vi "Load Subroutine Test Exec.vi"(4 "Path Builder":refnum<class "IPath Builder.lvclass">, 5 "Subroutine in":refnum<class "Subroutine.lvclass">, 6 "Persistence in":refnum<class "IPersist.lvclass">, 7 "Linked List ID":string, 8 "error in (no error)":errorcluster, 10 "Subroutine Path":path, 11 "Linked List Ref":refnum<data-value>) -> (0 "error out":errorcluster, 1 "Test File Version Match":bool, 2 "Test Executive Version Match":bool, 3 "Linked List Ref out":refnum<data-value>)   [LabVIEW 2017, in "Custom Type Test Executive.lvlib" / "Subroutine.lvclass"]
uses:
  <vilib>/gpm_packages/@cs/test-executive/Source/Custom Type Test Executive/Subroutine/Subroutine.lvclass
  <vilib>/gpm_packages/@cs/linked-list/Source/Linked List/ILinkedList/ILinked List.lvclass
  <vilib>/gpm_packages/@cs/persistence/source/IPersist/IPersist.lvclass
  <vilib>/gpm_packages/@cs/test-executive/Source/Path Builder/IPath Builder/IPath Builder.lvclass
  <vilib>/gpm_packages/@cs/test-executive/Source/Test Executive/ITestExecutive/ITest Executive.lvclass
  <vilib>/gpm_packages/@cs/test-executive/Source/Custom Type Test Executive/Test Executive Data Type/Test Executive.lvclass/Test Executive.ctl
  <vilib>/gpm_packages/@cs/data-type-serializer/source/Boolean/Boolean.lvclass/Boolean.ctl
  <vilib>/gpm_packages/@cs/test-executive/Source/Custom Type Test Executive/Custom Type Test Executive/Custom Type Test Executive.lvclass
  C:/Program Files/National Instruments/LabVIEW 2017/vi.lib/gpm_packages/@cs/test-executive/Source/Test Executive/ITestExecutive/ITest Executive.lvclass
  <vilib>/gpm_packages/@cs/data-type-serializer/source/String/String.lvclass/String.ctl
  8fd00299-f1f7-40b8-accc-d4ca8393805f.vi
  7c02b004-8b9d-45a5-be84-3e65cc974b1d.vi
  eeacede9-d011-4dba-942b-6df48e717fe6.vi
  82c2d36c-c725-40f4-a6f6-462dea4f116e.vi
  7a4b305b-7132-4b75-8629-811f3558ef42.vi
  cfb7364d-dae3-4f2b-ba87-61db7f054fd9.vi
  1f521296-bf4a-4187-b7fe-4ed0693accc0.vi
  b9c2613a-6aa9-4761-86d5-781f96568d67.vi
  <vilib>/gpm_packages/@cs/test-executive/Source/Custom Type Test Executive/Test Executive Data Type/Test Executive.lvclass
  C:/Program Files/National Instruments/LabVIEW 2017/vi.lib/gpm_packages/@cs/data-type-serializer/source/Data Type/Data Type.lvclass
  <vilib>/Utility/error.llb/Error Cluster From Error Code.vi
  <vilib>/gpm_packages/@cs/data-type-serializer/source/Boolean/Boolean.lvclass
  <vilib>/gpm_packages/@cs/data-type-serializer/source/String/String.lvclass
  <vilib>/gpm_packages/@cs/test-executive/Source/Test Executive/TestExecutive Ref/TestExecutive Ref.lvclass
  <vilib>/gpm_packages/@cs/linked-list/Source/Linked List/Linked List Ref/Linked List Ref.lvclass
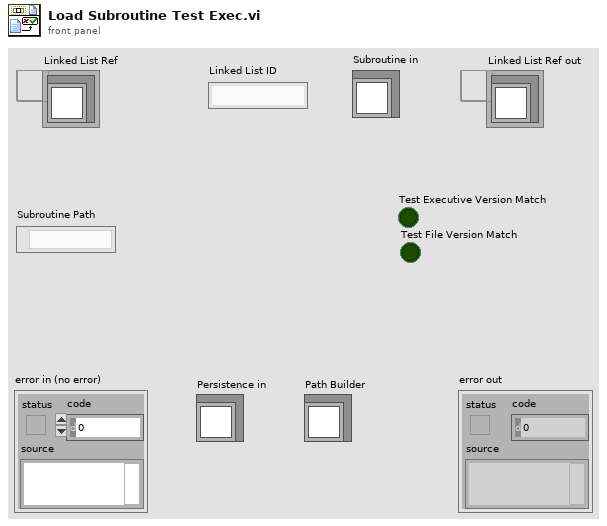
[diagram p1: front panel]
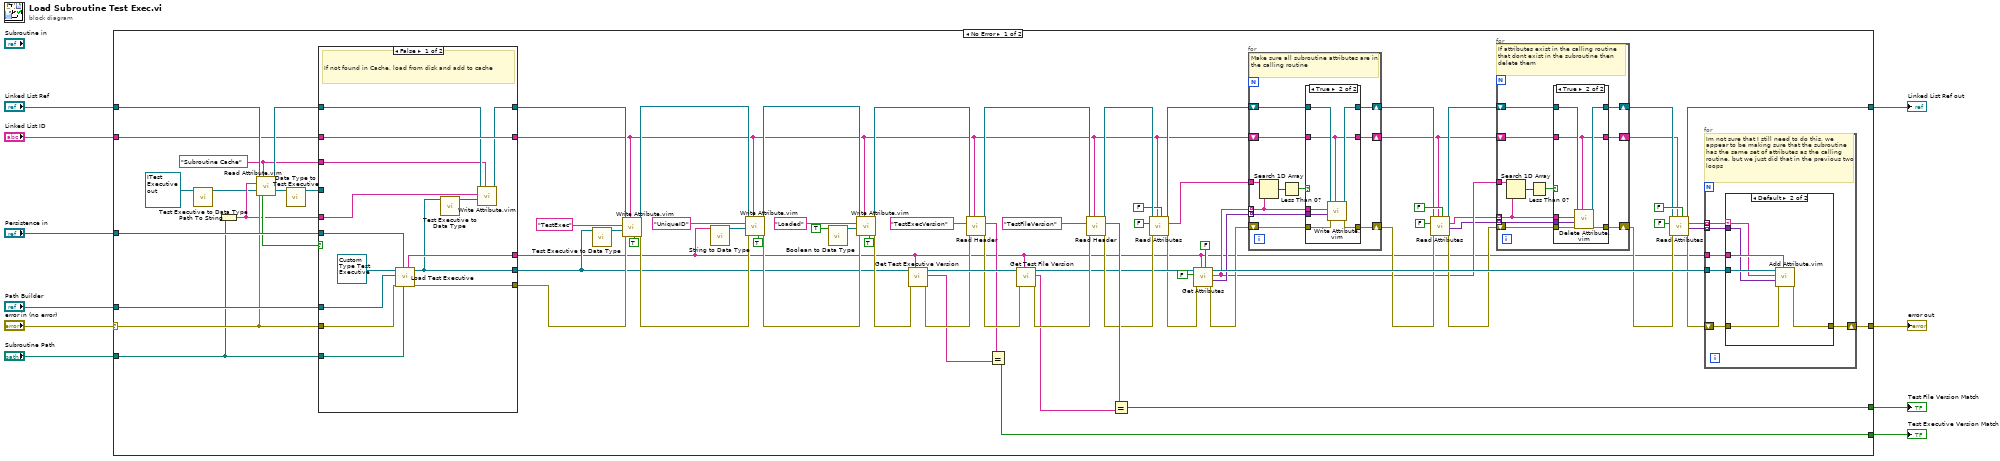
[diagram p0: block diagram]
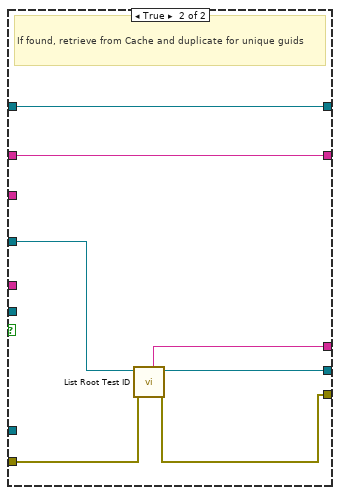
[diagram p2: hidden frame]
diagram:
  n1 = case shown="No Error" "error in (no error)" {
    selector: "error in (no error)" -> [w29 w168]
    tunnel: "Persistence in" -> [w82 _]
    tunnel: "Subroutine Path" -> [w28 _]
    tunnel: "Path Builder" -> [w81 _]
    tunnel: "Linked List Ref" -> [w30 w169]
    tunnel: [w65 _] -> w4
    tunnel: [w64 _] -> w3
    tunnel: "Linked List ID" -> [w24 _]
    tunnel: [w36 w169] -> w1
    tunnel: [w60 w168] -> w2
    frame No Error {
      w21 = "Subroutine Cache" ("Name")
      n2 = call <vilib>:"Test Executive to Data Type.vi"("Test Executive Ref"=refnum<data-value> refnum ("Test Executive Ref out")) -> ("Boolean out"=w19:refnum<class "Test Executive.lvclass">)  [unwired: 9 in, 1 out]
      n3 = Path To String(path=w28) -> (string=w22:string)
      n4 = call "Read Attribute.vim"("Linked List Ref"=w30, "Linked List ID"=w21, "Attribute Name"=w22, "Type"=w19, "error in (no error)"=w29) -> ("Linked List Ref out"=w26:refnum<data-value>, "Attribute"=w18:refnum<class "Test Executive.lvclass">, "Found?"=w27:bool)  [unwired: 5 in, 3 out]
      n5 = call <vilib>:"Data Type to Test Executive.vi"("Data Type"=w18) -> ("Test Executive Ref"=w17:refnum<data-value>)  [unwired: 9 in, 1 out]
      n6 = case shown="False" w27 {
        tunnel: [w105 w109] -> w87
        tunnel: w82 -> [w104 _]
        tunnel: w81 -> [w103 _]
        tunnel: [w94 w107] -> w15
        tunnel: [w95 w106] -> w13
        tunnel: w29 -> [w102 w110]
        tunnel: w28 -> [w101 _]
        tunnel: [w98 w112] -> w25
        tunnel: w26 -> [w99 w112]
        tunnel: [w100 w111] -> w23
        tunnel: w24 -> [w100 w111]
        tunnel: w22 -> [w96 _]
        tunnel: w21 -> [w97 _]
        tunnel: w17 -> [_ w108]
        frame False {
          # "If not found in Cache, load from disk and add to cache"
          n7 = call <vilib>:"Load Test Executive.vi"("Folder"=w101, "Persistence in"=w104, "error in (no error)"=w102, "Path Builder"=w103, "Test Executive"=refnum<class "Custom Type Test Executive.lvclass"> refnum ("Custom Type Test Executive.lvlib:Custom Type Test Executive.lvclass")) -> ("error out"=w105:errorcluster, "Test Executive Ref out"=w94:refnum<data-value>, "Root ID"=w95:string)  [unwired: 4 in]
          n8 = call <vilib>:"Test Executive to Data Type.vi"("Test Executive Ref"=w94) -> ("Boolean out"=w93:refnum<class "Test Executive.lvclass">)  [unwired: 9 in, 1 out]
          n9 = call "Write Attribute.vim"("Linked List ID"=w97, "Attribute"=w93, "Attribute Name"=w96, "Linked List Ref"=w99) -> ("Linked List Ref out"=w98:refnum<data-value>)  [unwired: 4 in, 3 out]
        }
        frame True {
          # "If found, retrieve from Cache and duplicate for unique guids"
          n10 = call <vilib>:"List Root Test ID.vi"("error in (no error)"=w110, "Test Executive Ref"=w108) -> ("error out"=w109:errorcluster, "Test Executive Ref out"=w107:refnum<data-value>, "Root ID"=w106:string)  [unwired: 5 in, 2 out]
        }
      }
      n11 = call <vilib>:"Test Executive to Data Type.vi"("Test Executive Ref"=w15) -> ("Boolean out"=w16:refnum<class "Test Executive.lvclass">)  [unwired: 9 in, 1 out]
      n12 = call "Write Attribute.vim"("Private?"=TRUE, "Linked List ID"=w23, "error in (no error)"=w87, "Attribute"=w16, "Attribute Name"="TestExec", "Linked List Ref"=w25) -> ("error out"=w88:errorcluster, "Linked List Ref out"=w80:refnum<data-value>)  [unwired: 2 in, 2 out]
      n13 = call <vilib>:"String to Data Type.vi"("String"=w13) -> ("Boolean out"=w14:refnum<class "String.lvclass">)  [unwired: 9 in, 1 out]
      n14 = call "Write Attribute.vim"("Private?"=TRUE, "Linked List ID"=w23, "error in (no error)"=w88, "Attribute"=w14, "Attribute Name"="UniqueID", "Linked List Ref"=w80) -> ("error out"=w84:errorcluster, "Linked List Ref out"=w79:refnum<data-value>)  [unwired: 2 in, 2 out]
      n15 = call <vilib>:"Boolean to Data Type.vi"("Boolean"=TRUE) -> ("Boolean out"=w12:refnum<class "Boolean.lvclass">)  [unwired: 9 in, 1 out]
      n16 = call "Write Attribute.vim"("Private?"=TRUE, "Linked List ID"=w23, "error in (no error)"=w84, "Attribute"=w12, "Attribute Name"="Loaded", "Linked List Ref"=w79) -> ("error out"=w77:errorcluster, "Linked List Ref out"=w76:refnum<data-value>)  [unwired: 2 in, 2 out]
      n17 = call <vilib>:"Get Test Executive Version.vi"("Unique ID"=w13, "error in (no error)"=w77, "Test Executive Ref"=w15) -> ("error out"=w74:errorcluster, "Test Executive Version"=w68:string, "Test Executive Ref out"=w78:refnum<data-value>)  [unwired: 5 in, 1 out]
      n18 = call <vilib>:"Read Header.vi"("Linked List ID"=w23, "error in (no error)"=w74, "Header Name"="TestExecVersion" ("String"), "Linked List Ref"=w76) -> ("error out"=w73:errorcluster, "Header Value"=w69:string, "Linked List Ref out"=w72:refnum<data-value>)  [unwired: 4 in, 1 out]
      n19 = Equal?(x=w69, y=w68) -> (x = y?=w65:bool)
      n20 = call <vilib>:"Get Test File Version.vi"("Unique ID"=w13, "error in (no error)"=w73, "Test Executive Ref"=w78) -> ("error out"=w71:errorcluster, "Test File Version"=w66:string, "Test Executive Ref out"=w58:refnum<data-value>)  [unwired: 5 in, 1 out]
      n21 = call <vilib>:"Read Header.vi"("Linked List ID"=w23, "error in (no error)"=w71, "Header Name"="TestFileVersion" ("String"), "Linked List Ref"=w72) -> ("error out"=w62:errorcluster, "Header Value"=w67:string, "Linked List Ref out"=w63:refnum<data-value>)  [unwired: 4 in, 1 out]
      n22 = Equal?(x=w67, y=w66) -> (x = y?=w64:bool)
      n23 = call <vilib>:"Read Attributes.vi"("Flatten Pointer?"=FALSE, "Linked List ID"=w23, "error in (no error)"=w62, "Include Private?"=FALSE, "Linked List Ref"=w63) -> ("error out"=w54:errorcluster, "Attribute Names out"=w53:string[], "Linked List Ref out"=w51:refnum<data-value>)  [unwired: 1 in, 3 out]
      n24 = call <vilib>:"Get Attributes.vi"("Flatten Pointer?"=FALSE, "Test ID"=w13, "error in (no error)"=w54, "Include Private?"=FALSE, "Test Executive Ref"=w58) -> ("error out"=w50:errorcluster, "Attributes"=w52:variant[], "Attribute Names out"=w42:string[], "Test Executive Ref out"=w57:refnum<data-value>)  [unwired: 1 in, 2 out]
      n25 = for {
        tunnel: w42 -> [w136] mode=indexing
        tunnel: w52 -> [w135] mode=indexing
        shift-right: [w141] -> w46
        shift-left: w51 -> [w142]
        tunnel: w53 -> [w143]
        shift-right: [w139] -> w47
        shift-left: w50 -> [w140]
        shift-right: [w134] -> w44
        shift-left: w23 -> [w138]
        # "Make sure all subroutine attributes are in the calling routine"
        n26 = Search 1D Array(1D array=w143, element=w136) -> (index of element=w144:i32)  [unwired: 1 in]
        n27 = Less Than 0?(x=w144) -> (x < 0?=w137:bool)
        n28 = case shown="True" w137 {
          tunnel: w142 -> [w147 w154]
          tunnel: [w147 w153] -> w141
          tunnel: w140 -> [w146 w152]
          tunnel: [w146 w151] -> w139
          tunnel: w138 -> [w145 w148]
          tunnel: w136 -> [_ w150]
          tunnel: w135 -> [_ w149]
          tunnel: [w145 w148] -> w134
          frame False {
          }
          frame True {
            n29 = call "Write Attribute.vim"("Linked List ID"=w148, "error in (no error)"=w152, "Attribute"=w149, "Attribute Name"=w150, "Linked List Ref"=w154) -> ("error out"=w151:errorcluster, "Linked List Ref out"=w153:refnum<data-value>)  [unwired: 3 in, 2 out]
          }
        }
      }
      n30 = call <vilib>:"Read Attributes.vi"("Flatten Pointer?"=FALSE, "Linked List ID"=w44, "error in (no error)"=w47, "Include Private?"=FALSE, "Linked List Ref"=w46) -> ("error out"=w43:errorcluster, "Attributes"=w40:variant[], "Attribute Names out"=w41:string[], "Linked List Ref out"=w45:refnum<data-value>)  [unwired: 1 in, 2 out]
      n31 = for {
        tunnel: w41 -> [w115] mode=indexing
        tunnel: w40 -> [w114] mode=indexing
        shift-right: [w120] -> w37
        shift-left: w45 -> [w121]
        tunnel: w42 -> [w122]
        shift-right: [w118] -> w34
        shift-left: w43 -> [w119]
        shift-right: [w113] -> w35
        shift-left: w44 -> [w117]
        # "If attributes exist in the calling routine that dont exist in the subroutine then delete them"
        n32 = Search 1D Array(1D array=w122, element=w115) -> (index of element=w123:i32)  [unwired: 1 in]
        n33 = Less Than 0?(x=w123) -> (x < 0?=w116:bool)
        n34 = case shown="True" w116 {
          tunnel: w121 -> [w126 w133]
          tunnel: [w126 w132] -> w120
          tunnel: w119 -> [w125 w130]
          tunnel: [w125 w129] -> w118
          tunnel: w117 -> [w124 w131]
          tunnel: w115 -> [_ w128]
          tunnel: w114 -> [_ w127]
          tunnel: [w124 w131] -> w113
          frame False {
          }
          frame True {
            n35 = call "Delete Attribute.vim"("Linked List ID"=w131, "error in (no error)"=w130, "Type"=w127, "Attribute Name"=w128, "Linked List Ref"=w133) -> ("error out"=w129:errorcluster, "Linked List Ref out"=w132:refnum<data-value>)  [unwired: 4 in, 1 out]
          }
        }
      }
      n36 = call <vilib>:"Read Attributes.vi"("Flatten Pointer?"=FALSE, "Linked List ID"=w35, "error in (no error)"=w34, "Include Private?"=FALSE, "Linked List Ref"=w37) -> ("error out"=w33:errorcluster, "Attributes"=w32:variant[], "Attribute Names out"=w31:string[], "Linked List Ref out"=w36:refnum<data-value>)  [unwired: 1 in, 2 out]
      n37 = for {
        tunnel: w57 -> [w160]
        tunnel: w13 -> [w159]
        shift-right: [w157] -> w60
        shift-left: w33 -> [w158]
        tunnel: w31 -> [w156] mode=indexing
        tunnel: w32 -> [w155] mode=indexing
        # "Im not sure that I still need to do this, we appear to be making sure that the subroutine has the same set of attributes as the calling routine, but we just did that in the previous two loops"
        n38 = case shown="Default" w156 {
          selector: w156 -> [_ w163]
          tunnel: w160 -> [_ w167]
          tunnel: w159 -> [_ w166]
          tunnel: w158 -> [w161 w165]
          tunnel: [w161 w164] -> w157
          tunnel: w155 -> [_ w162]
          frame "Restore Point" {
          }
          frame Default {
            n39 = call "Add Attribute.vim"("ID"=w166, "error in (no error)"=w165, "Attribute"=w162, "Attribute Name"=w163, "Test Executive Ref"=w167) -> ("error out"=w164:errorcluster)  [unwired: 3 in, 3 out]
          }
        }
      }
    }
    frame Error {
    }
  }
  "error out" <- w2
  "Linked List Ref out" <- w1
  "Test Executive Version Match" <- w4
  "Test File Version Match" <- w3
